vi "WriteConfig.vi"(8 "error in (no error)":errorcluster, 10 "Config":variant, 11 "SiemensDigitalEnergyMeter in":refnum<class "SiemensDigitalEnergyMeter.lvclass">) -> (0 "error out":errorcluster, 3 "SiemensDigitalEnergyMeter out":refnum<class "SiemensDigitalEnergyMeter.lvclass">)   [LabVIEW 2018, in "SensorPlugins.lvlib" / "SiemensDigitalEnergyMeter.lvclass"]
doc: "This VI unpacks the configuration information transmitted and updates the relevant cluster with this information."
uses:
  SiemensDigitalEnergyMeter.lvclass
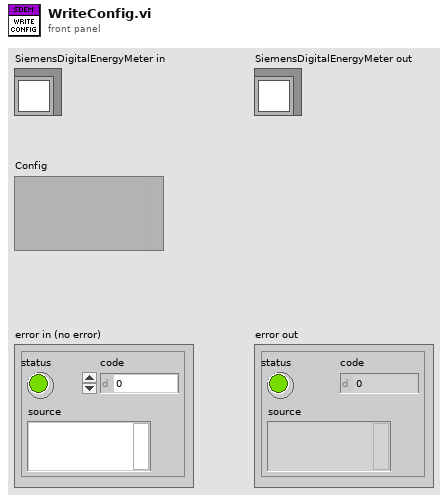
[diagram p1: front panel]
types:
  T1 = typedef "SensorPlugins.lvlib/SiemensDigitalEnergyMeter.lvclass/MeasurementControls.ctl" = cluster{"Measurement RefreshTime (ms)":u32, "Measurement Name":string}
  T2 = typedef "SensorPlugins.lvlib/SiemensDigitalEnergyMeter.lvclass/SiemensDigitalEnergyMeterControls.ctl" = cluster{"Measurement(s)":u16[], "Configuration Commands":string, "Use Measurement Commands Text Box?":bool, "Measurement Commands":string, "Connected?":bool, "Serial Number":string, "IP Address":string, "Port (502)":u16, "Unit ID":u8, "Serial Type":enum16{"RTU", "ASCII"}, "Using TCP?":bool, "VISA Resource Name":string}[]
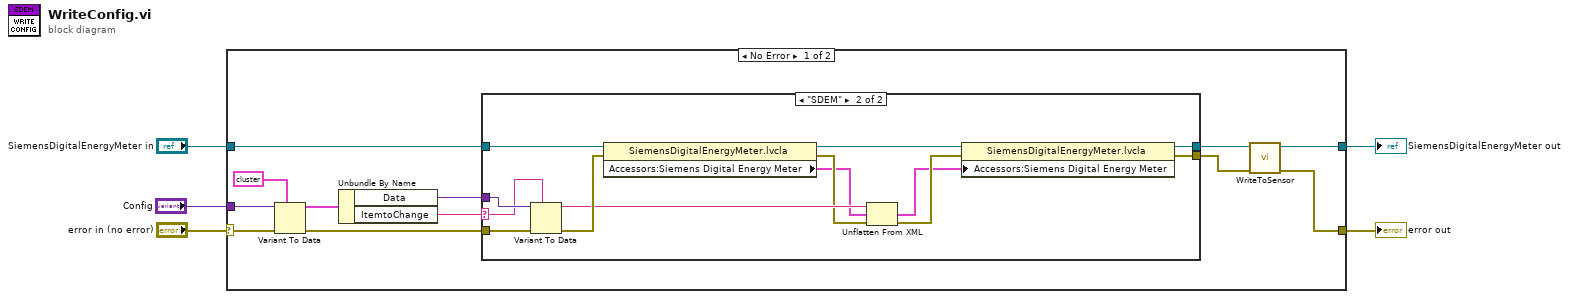
[diagram p0: block diagram]
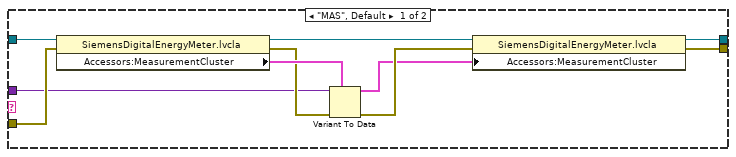
[diagram p2: hidden frame]
diagram:
  n1 = case shown="No Error" "error in (no error)" {
    selector: "error in (no error)" -> [w15 w42]
    tunnel: [w8 w42] -> w4
    tunnel: "SiemensDigitalEnergyMeter in" -> [w17 w41]
    tunnel: [w6 w41] -> w2
    tunnel: "Config" -> [w16 _]
    frame No Error {
      n2 = Variant To Data(error in=w15, type=cluster{"Data":variant, "ItemtoChange":string} {"Data"=variant, "ItemtoChange"=""}, Variant=w16) -> (data=w12:cluster{"Data":variant, "ItemtoChange":string}, error out=w14:errorcluster)
      n3 = Unbundle By Name(w12) -> ("Data"=w11:variant, "ItemtoChange"=w10:string)
      n4 = case shown="\"SDEM\"" w10 {
        selector: w10 -> [_ w33]
        tunnel: w17 -> [w27 w40]
        tunnel: [w25 w38] -> w7
        tunnel: [w24 w37] -> w9
        tunnel: w14 -> [w23 w35]
        tunnel: w11 -> [w20 w36]
        frame "MAS", Default {
          n5 = property class="SiemensDigitalEnergyMeter.lvcla"(reference=w27, error in=w23) -> (reference out=w26:refnum<class "SiemensDigitalEnergyMeter.lvclass">, error out=w21:errorcluster, "Accessors:MeasurementCluster"=w22:T1)
          n6 = Variant To Data(error in=w21, type=w22, Variant=w20) -> (data=w18:T1, error out=w19:errorcluster)
          n7 = property class="SiemensDigitalEnergyMeter.lvcla"(reference=w26, error in=w19, "Accessors:MeasurementCluster"=w18) -> (reference out=w25:refnum<class "SiemensDigitalEnergyMeter.lvclass">, error out=w24:errorcluster)
        }
        frame "SDEM" {
          n8 = Variant To Data(error in=w35, type=w33, Variant=w36) -> (data=w32:string, error out=w34:errorcluster)
          n9 = property class="SiemensDigitalEnergyMeter.lvcla"(reference=w40, error in=w34) -> (reference out=w39:refnum<class "SiemensDigitalEnergyMeter.lvclass">, error out=w31:errorcluster, "Accessors:Siemens Digital Energy Meter"=w30:T2)
          n10 = Unflatten From XML(xml string=w32, type=w30, error in (no error)=w31) -> (value=w28:T2, error out=w29:errorcluster)
          n11 = property class="SiemensDigitalEnergyMeter.lvcla"(reference=w39, error in=w29, "Accessors:Siemens Digital Energy Meter"=w28) -> (reference out=w38:refnum<class "SiemensDigitalEnergyMeter.lvclass">, error out=w37:errorcluster)
        }
      }
      n12 = call-dynamic "WriteToSensor.vi"("error in (no error)"=w9, "SiemensDigitalEnergyMeter in"=w7) -> ("error out"=w8:errorcluster, "SiemensDigitalEnergyMeter out"=w6:refnum<class "SiemensDigitalEnergyMeter.lvclass">)  [unwired: 8 in]
    }
    frame Error {
    }
  }
  "error out" <- w4
  "SiemensDigitalEnergyMeter out" <- w2
